vi "NI 9265_DOUBLETASK_AO.vi"(8 "error in":errorcluster, 10 "MODULE NAME 2":string="CDR_AO2", 11 "MODULE NAME":string="CDR_AO1") -> (0 "error out":errorcluster, 3 "task out":refnum<k21>)   [LabVIEW 2016]
uses:
  <vilib>/DAQmx/create/channels.llb/DAQmx Create Channel (AO-Current-Basic).vi
  <resource>/objmgr/daqmx.rc
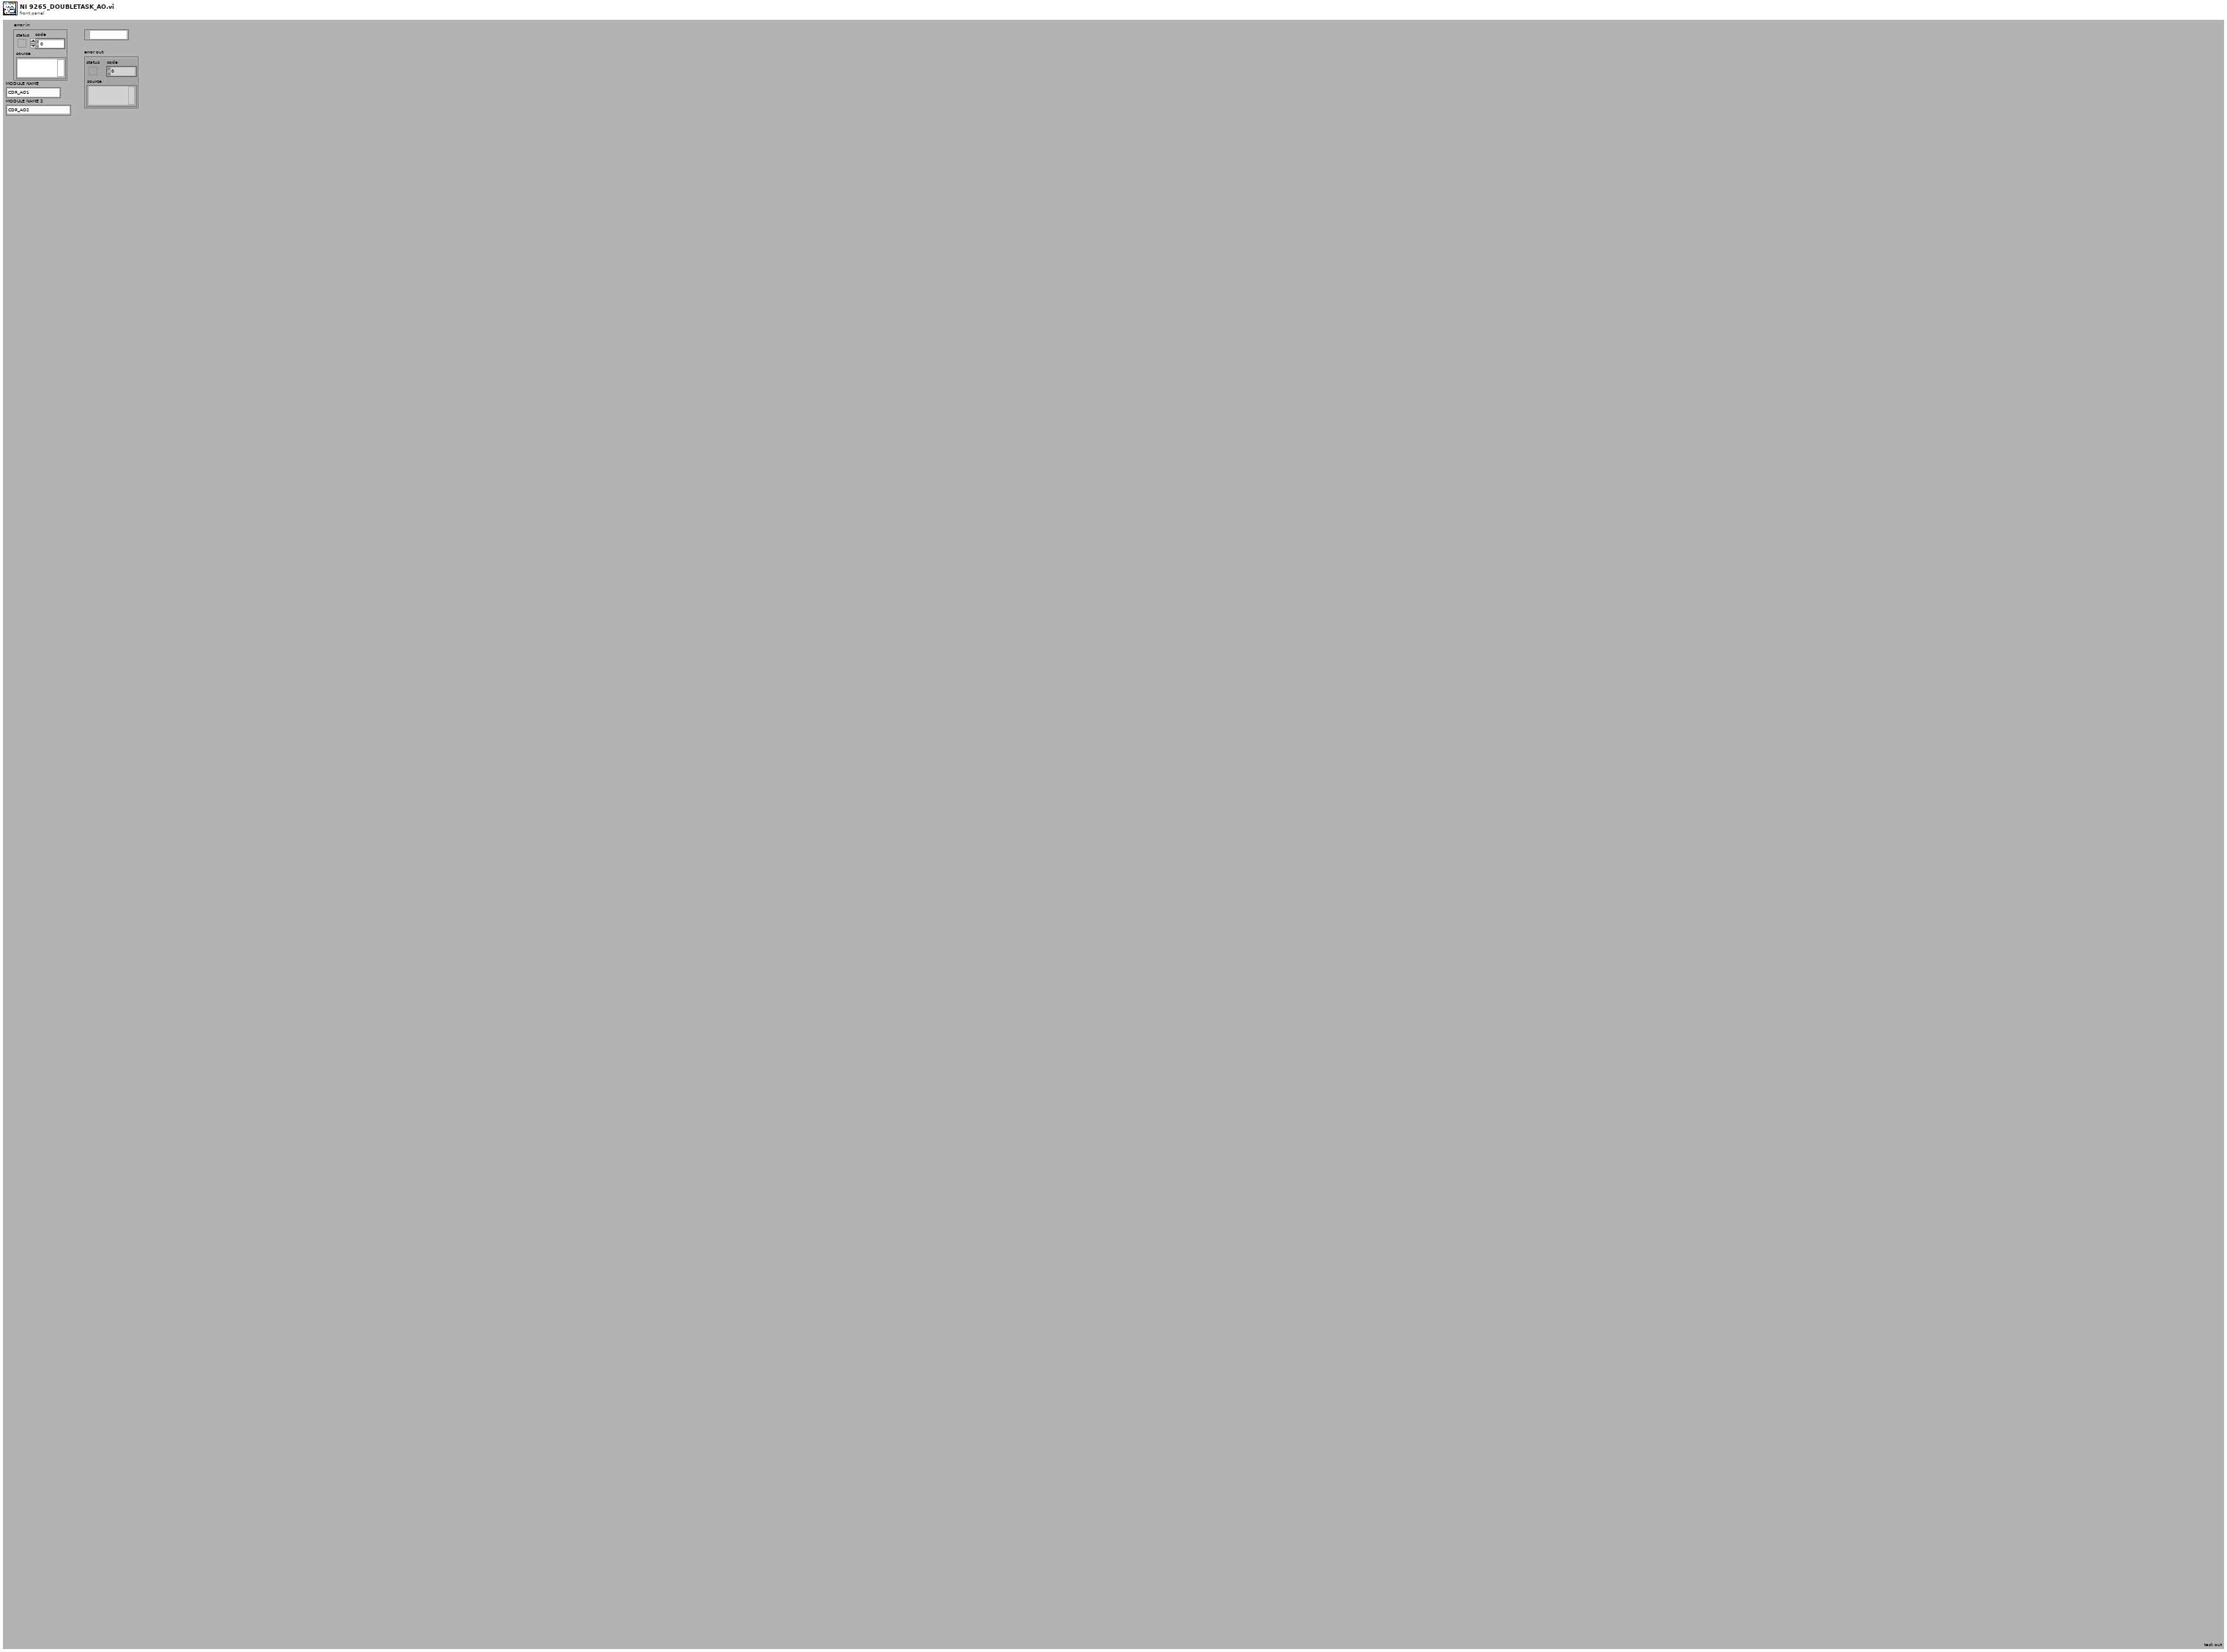
[diagram p1: front panel]
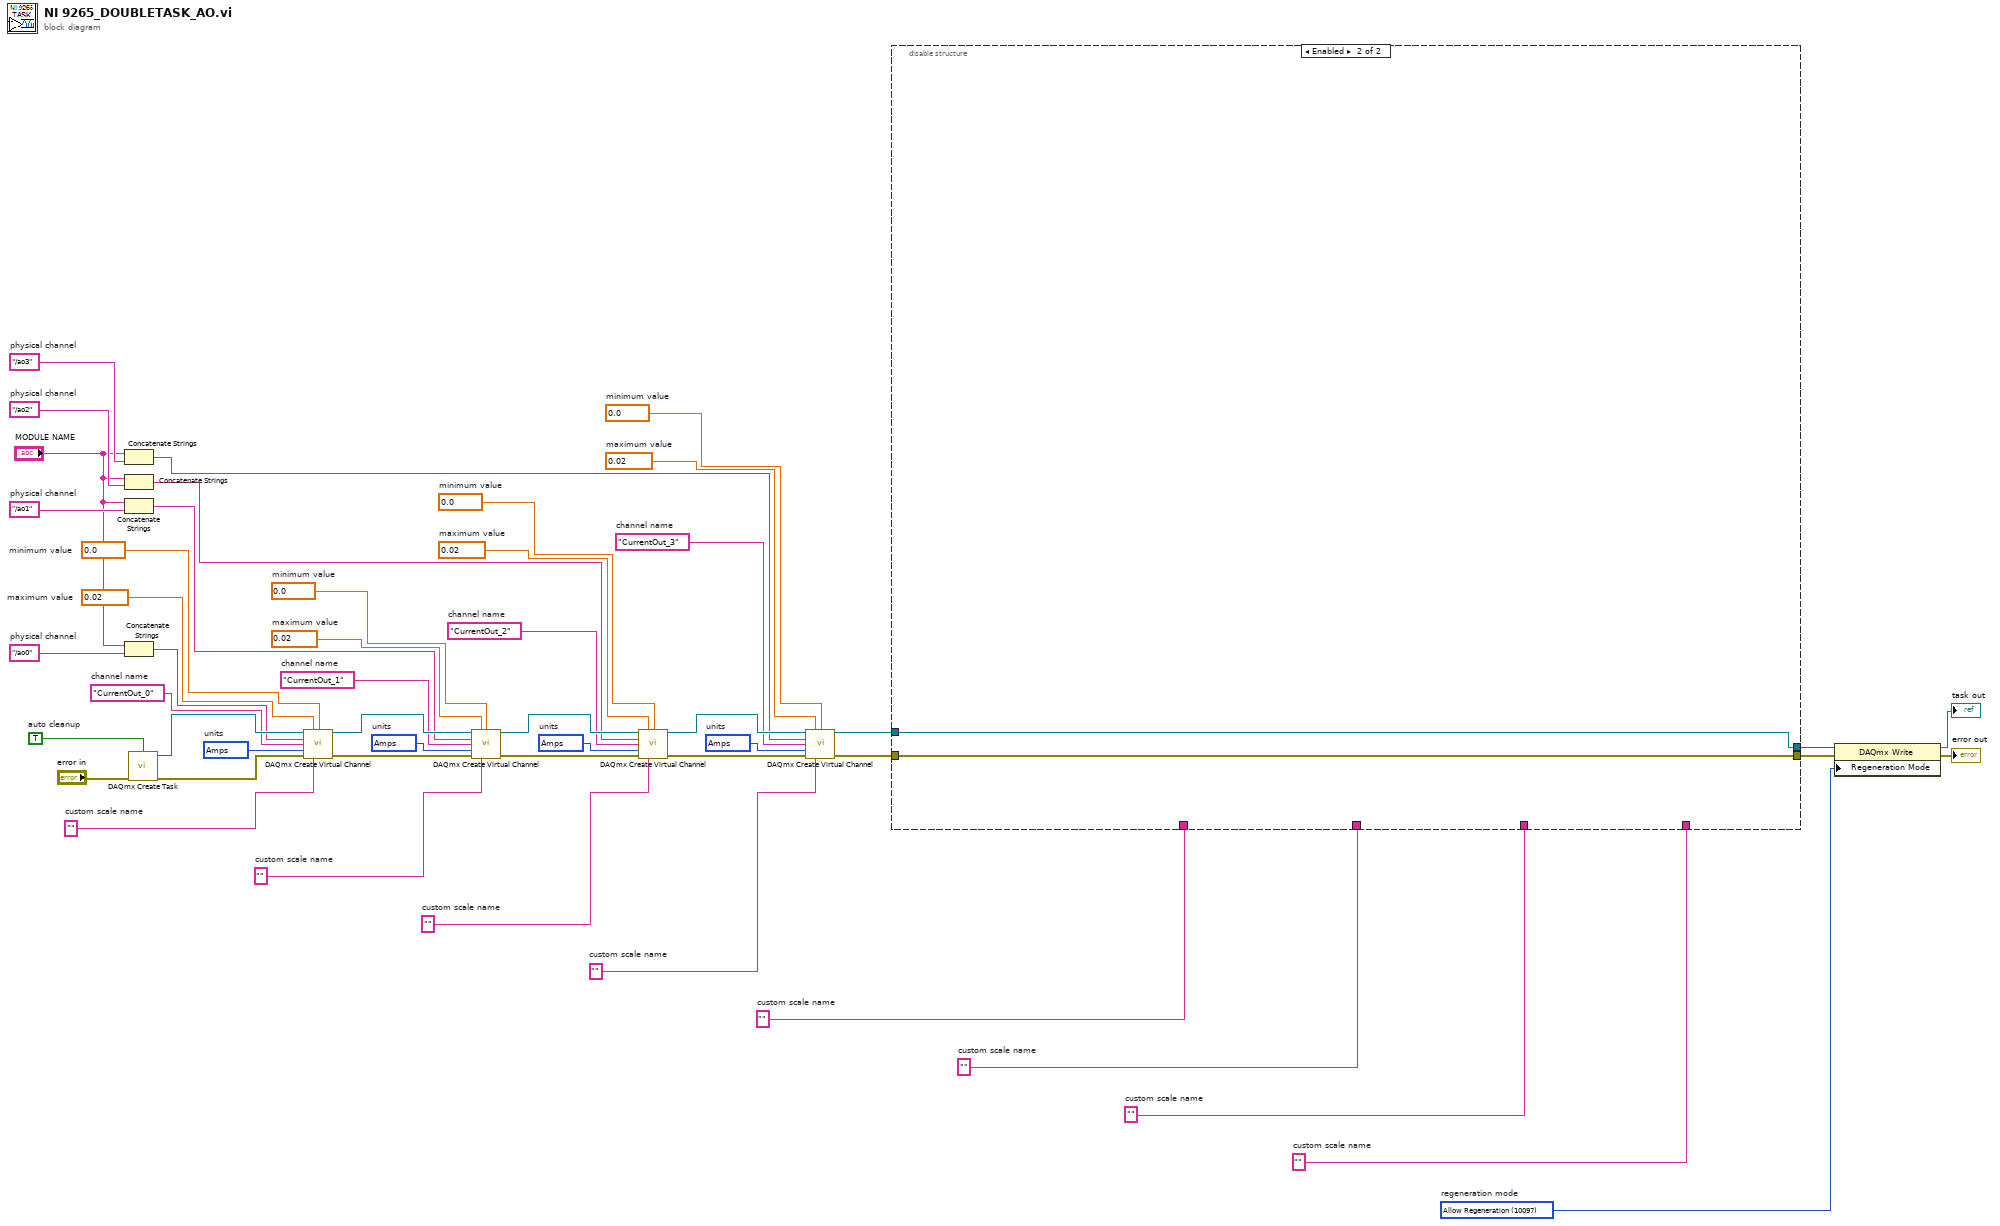
[diagram p0: block diagram]
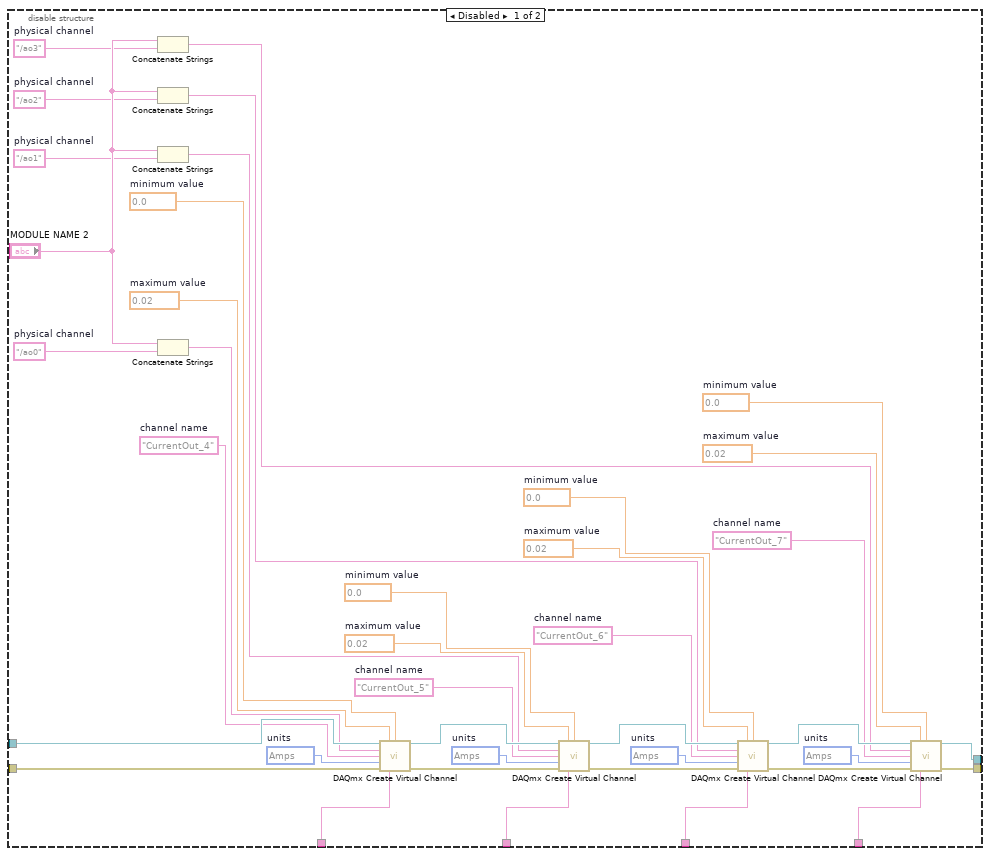
[diagram p2: hidden frame]
diagram:
  w14 = 10097 items=["Allow Regeneration"=10097, "Do Not Allow Regeneration"=10158]  # regeneration mode
  w15 = ""  # custom scale name
  w16 = ""  # custom scale name
  w17 = ""  # custom scale name
  w18 = ""  # custom scale name
  w20 = 10342 items=["Amps"=10342, "From Custom Scale"=10065]  # units
  w21 = "CurrentOut_3"  # channel name
  w23 = ""  # custom scale name
  w24 = 0.0  # minimum value
  w25 = 0.02  # maximum value
  w4 = "/ao3"  # physical channel
  w27 = 10342 items=["Amps"=10342, "From Custom Scale"=10065]  # units
  w28 = "CurrentOut_2"  # channel name
  w30 = ""  # custom scale name
  w31 = 0.0  # minimum value
  w32 = 0.02  # maximum value
  w6 = "/ao2"  # physical channel
  w34 = 10342 items=["Amps"=10342, "From Custom Scale"=10065]  # units
  w35 = "CurrentOut_1"  # channel name
  w37 = ""  # custom scale name
  w38 = 0.0  # minimum value
  w39 = 0.02  # maximum value
  w7 = "/ao1"  # physical channel
  w41 = 10342 items=["Amps"=10342, "From Custom Scale"=10065]  # units
  w42 = "CurrentOut_0"  # channel name
  w44 = ""  # custom scale name
  w45 = 0.0  # minimum value
  w46 = 0.02  # maximum value
  w9 = "/ao0"  # physical channel
  w48 = TRUE  # auto cleanup
  n1 = Concatenate Strings("MODULE NAME", w4) -> (w3:string)
  n2 = Concatenate Strings("MODULE NAME", w6) -> (w5:string)
  n3 = Concatenate Strings("MODULE NAME", w7) -> (w2:string)
  n4 = Concatenate Strings("MODULE NAME", w9) -> (w8:string)
  n5 = call <vilib>:"DAQmx Create Task.vi"("auto cleanup"=w48, "error in"="error in") -> ("task out"=w47:refnum<k21>, "error out"=w49:errorcluster)  [unwired: 12 in]
  n6 = call-poly <vilib>:"DAQmx Create Virtual Channel.vi"("task in"=w47, "maximum value"=w46, "minimum value"=w45, "physical channels"=w8, "name to assign"=w42, "units"=w41, "error in"=w49, "custom scale name"=w44) -> ("task out"=w40:refnum<k21>, "error out"=w43:errorcluster)  [unwired: 6 in]
  n7 = call-poly <vilib>:"DAQmx Create Virtual Channel.vi"("task in"=w40, "maximum value"=w39, "minimum value"=w38, "physical channels"=w2, "name to assign"=w35, "units"=w34, "error in"=w43, "custom scale name"=w37) -> ("task out"=w33:refnum<k21>, "error out"=w36:errorcluster)  [unwired: 6 in]
  n8 = call-poly <vilib>:"DAQmx Create Virtual Channel.vi"("task in"=w33, "maximum value"=w32, "minimum value"=w31, "physical channels"=w5, "name to assign"=w28, "units"=w27, "error in"=w36, "custom scale name"=w30) -> ("task out"=w26:refnum<k21>, "error out"=w29:errorcluster)  [unwired: 6 in]
  n9 = call-poly <vilib>:"DAQmx Create Virtual Channel.vi"("task in"=w26, "maximum value"=w25, "minimum value"=w24, "physical channels"=w3, "name to assign"=w21, "units"=w20, "error in"=w29, "custom scale name"=w23) -> ("task out"=w19:refnum<k21>, "error out"=w22:errorcluster)  [unwired: 6 in]
  n10 = disable-structure shown="Enabled" {
    disable-tunnel: w22 -> [w89 w90]
    disable-tunnel: w19 -> [w88 w91]
    disable-tunnel: w18 -> [w85 _]
    disable-tunnel: w17 -> [w78 _]
    disable-tunnel: w16 -> [w71 _]
    disable-tunnel: w15 -> [w64 _]
    disable-tunnel: [w61 w91] -> w11
    disable-tunnel: [w60 w90] -> w10
    frame Disabled {
      w62 = 10342 items=["Amps"=10342, "From Custom Scale"=10065]  # units
      w63 = "CurrentOut_7"  # channel name
      w65 = 0.0  # minimum value
      w66 = 0.02  # maximum value
      w52 = "/ao3"  # physical channel
      w68 = 10342 items=["Amps"=10342, "From Custom Scale"=10065]  # units
      w69 = "CurrentOut_6"  # channel name
      w72 = 0.0  # minimum value
      w73 = 0.02  # maximum value
      w54 = "/ao2"  # physical channel
      w75 = 10342 items=["Amps"=10342, "From Custom Scale"=10065]  # units
      w76 = "CurrentOut_5"  # channel name
      w79 = 0.0  # minimum value
      w80 = 0.02  # maximum value
      w56 = "/ao1"  # physical channel
      w82 = 10342 items=["Amps"=10342, "From Custom Scale"=10065]  # units
      w83 = "CurrentOut_4"  # channel name
      w86 = 0.0  # minimum value
      w87 = 0.02  # maximum value
      w58 = "/ao0"  # physical channel
      n11 = Concatenate Strings("MODULE NAME 2", w52) -> (w51:string)
      n12 = Concatenate Strings("MODULE NAME 2", w54) -> (w53:string)
      n13 = Concatenate Strings("MODULE NAME 2", w56) -> (w55:string)
      n14 = Concatenate Strings("MODULE NAME 2", w58) -> (w57:string)
      n15 = call-poly <vilib>:"DAQmx Create Virtual Channel.vi"("task in"=w88, "maximum value"=w87, "minimum value"=w86, "physical channels"=w57, "name to assign"=w83, "units"=w82, "error in"=w89, "custom scale name"=w85) -> ("task out"=w81:refnum<k21>, "error out"=w84:errorcluster)  [unwired: 6 in]
      n16 = call-poly <vilib>:"DAQmx Create Virtual Channel.vi"("task in"=w81, "maximum value"=w80, "minimum value"=w79, "physical channels"=w55, "name to assign"=w76, "units"=w75, "error in"=w84, "custom scale name"=w78) -> ("task out"=w74:refnum<k21>, "error out"=w77:errorcluster)  [unwired: 6 in]
      n17 = call-poly <vilib>:"DAQmx Create Virtual Channel.vi"("task in"=w74, "maximum value"=w73, "minimum value"=w72, "physical channels"=w53, "name to assign"=w69, "units"=w68, "error in"=w77, "custom scale name"=w71) -> ("task out"=w67:refnum<k21>, "error out"=w70:errorcluster)  [unwired: 6 in]
      n18 = call-poly <vilib>:"DAQmx Create Virtual Channel.vi"("task in"=w67, "maximum value"=w66, "minimum value"=w65, "physical channels"=w51, "name to assign"=w63, "units"=w62, "error in"=w70, "custom scale name"=w64) -> ("task out"=w61:refnum<k21>, "error out"=w60:errorcluster)  [unwired: 6 in]
    }
    frame Enabled {
    }
  }
  n19 = property class="DAQmx Write"(reference=w11, error in=w10, "Regeneration Mode"=w14) -> (reference out=→"task out":refnum<k21>, error out=→"error out":errorcluster)
